vi "PDF CG Test Spans inaktiv setzen.vi"() -> (1 "Span 3":bool, 2 "Span 2":bool, 3 "Span 1":bool)   [LabVIEW 2020, in "Erweiterte Konfig.lvlib" / "CG-Check Konfig.lvlib"]
uses:
  CG-Check Konfig.lvlib
  Schedule Modul/Aktion FGV Testdaten sammeln.ctl
  Schedule Modul/Schedule Modul.lvlib
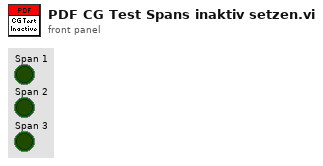
[diagram p1: front panel]
types:
  T1 = typedef "Schedule Modul.lvlib/Aktion FGV Testdaten sammeln.ctl" = enum16{"lesen", "Dichtheitstest", "CalGasTest", "T90", "Kalibrieren", "init", "Kalender Daten"}
  T2 = typedef "Schedule Modul.lvlib/Ergebnis CalGas Test.ctl" = cluster{"Istwerte":string[][], "Auswertung":string[][][], "Fehler":bool[], "Abweichung in %":string[][], "Spanauswahl":i32[]}
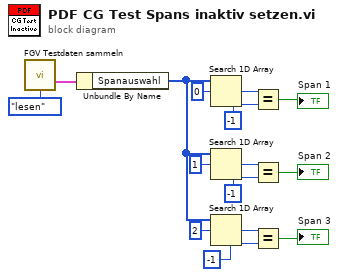
[diagram p0: block diagram]
diagram:
  n1 = call "FGV Testdaten sammeln.vi"("Aktion"=Aktion_FGV_Testdaten_sammeln."lesen") -> ("Ergebnis CalGas Test"=w4:T2)  [unwired: 9 in, 5 out]
  n2 = Unbundle By Name(w4) -> ("Spanauswahl"=w12:i32[])
  n3 = Search 1D Array(1D array=w12, element=0 ("Element")) -> (index of element=w6:i32)  [unwired: 1 in]
  n4 = Search 1D Array(1D array=w12, element=1 ("Element")) -> (index of element=w9:i32)  [unwired: 1 in]
  n5 = Search 1D Array(1D array=w12, element=2 ("Element")) -> (index of element=w10:i32)  [unwired: 1 in]
  n6 = Equal?(x=w6, y=-1) -> (x = y?=→"Span 1":bool)
  n7 = Equal?(x=w9, y=-1) -> (x = y?=→"Span 2":bool)
  n8 = Equal?(x=w10, y=-1) -> (x = y?=→"Span 3":bool)
